vi "本地数字信号仿真 - 副本.vi"() -> ()   [LabVIEW 2012]
uses:
  <vilib>/ptbypt/Frequency Domain.llb/Real FFT PtByPt.vi
  <vilib>/ptbypt/NI_PtbyPt.lvlib
  <vilib>/Analysis/NI_AALBase.lvlib
panel:
  out "Last Element Inserted 3.78MHz":dbl caption="最后插入的元素" format="%0.2f"
  out "Last Element Removed 3.78MHz":dbl caption="最后删除的元素" format="%0.2f"
  out "Last Element Inserted":dbl caption="最后插入的元素" format="%0.2f"
  out "Last Element Removed":dbl caption="最后删除的元素" format="%0.2f"
  out "Elements in Queue":i32(slide) caption="队列中的元素" scale=0.0..60000000.0 scale format="%0.0f"
  out "Waveform Chart":cluster{"Last Element Inserted":dbl, dbl}(graph) caption="波形图表"
  out "Elements in Queue 2":i32(slide) caption="队列中的元素" scale=0.0..60000000.0 scale format="%0.0f"
  out "Waveform Chart 2":cluster{"Last Element Inserted":dbl, dbl}(graph) caption="波形图表"
  in  "Queue Size":i32=60000000 caption="队列大小"
  in  "停止":bool
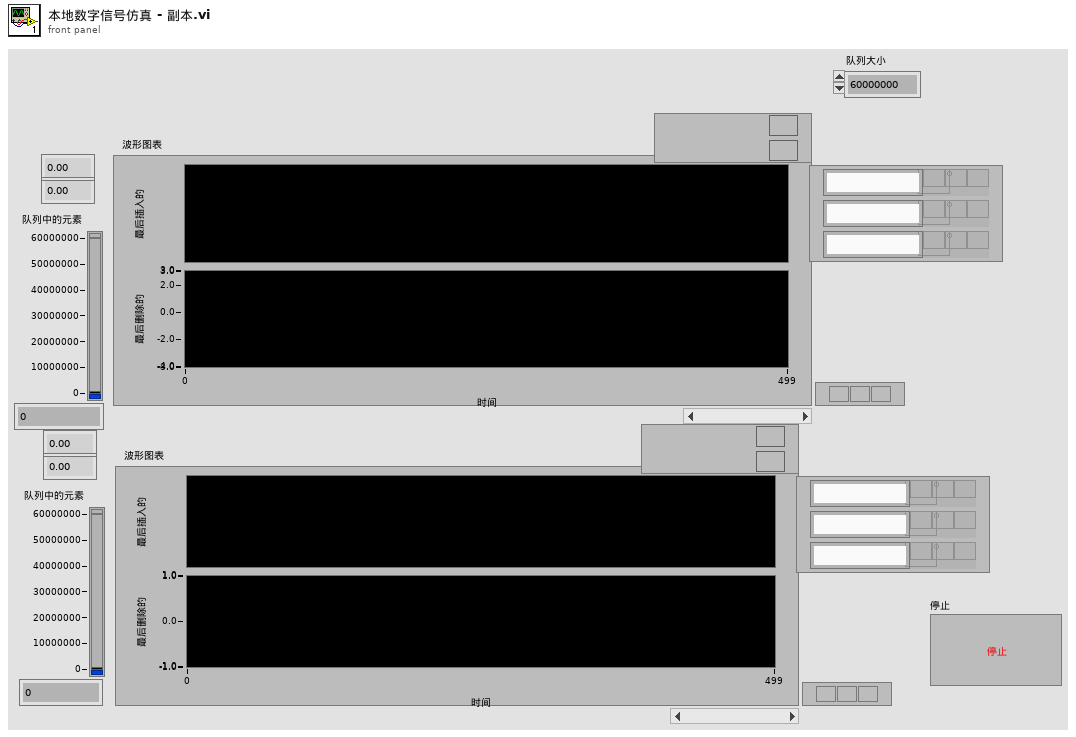
[diagram p1: front panel]
types:
  T1 = cluster{"Last Element Inserted":dbl, "Last Element Removed":dbl}
  T2 = cluster{"Last Element Inserted 3.78MHz":dbl, "Last Element Removed 3.78MHz":dbl}
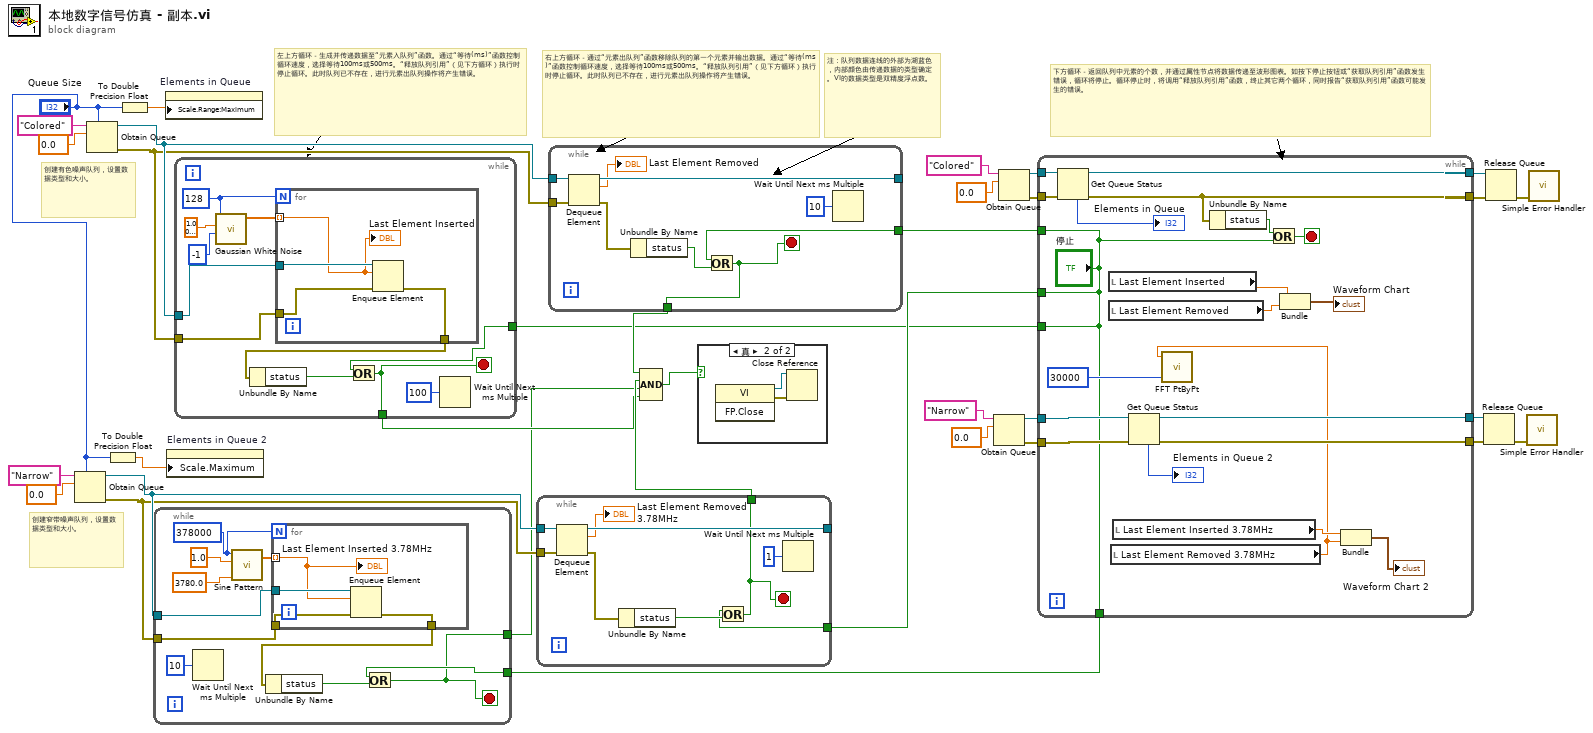
[diagram p0: block diagram]
diagram:
  # "创建窄带噪声队列，设置数据类型和大小。"
  # "右上方循环－通过“元素出队列”函数移除队列的第一个元素并输出数据。通过“等待(ms)”函数控制循环速度，选择等待100ms或500ms。“释放队列引用”（见下方循环）执行时停止循环。此时队列已不存在，进行元素出队列操作将产生错误。"
  # "注：队列数据连线的外部为湖蓝色，内部颜色由传递数据的类型确定。VI的数据类型是双精度浮点数。"
  # "下方循环－返回队列中元素的个数，并通过属性节点将数据传递至波形图表。如按下停止按钮或“获取队列引用”函数发生错误，循环将停止。循环停止时，将调用“释放队列引用”函数，终止其它两个循环，同时报告“获取队列引用”函数可能发生的错误。"
  # "左上方循环－生成并传递数据至“元素入队列”函数。通过“等待(ms)”函数控制循环速度，选择等待100ms或500ms。“释放队列引用”（见下方循环）执行时停止循环。此时队列已不存在，进行元素出队列操作将产生错误。"
  # "创建有色噪声队列，设置数据类型和大小。"
  n1 = Obtain Queue(max queue size (-1, unlimited)="Queue Size", name (unnamed)="Narrow", element data type=0.0) -> (queue out=w22:refnum<queue>, error out=w21:errorcluster)  [unwired: 2 in, 1 out]
  n2 = Obtain Queue(max queue size (-1, unlimited)="Queue Size", name (unnamed)="Colored", element data type=0.0) -> (queue out=w26:refnum<queue>, error out=w25:errorcluster)  [unwired: 2 in, 1 out]
  n3 = To Double Precision Float(number="Queue Size") -> (double precision float=w20:dbl)
  n4 = To Double Precision Float(number="Queue Size") -> (double precision float=w34:dbl)
  n5 = property on="Elements in Queue" class="Slide (严格)"("Scale.Range:Maximum"=w34) -> ()  [unwired: 2 in, 2 out]
  n6 = property on="Elements in Queue 2" class="Slide (严格)"("Scale.Maximum"=w20) -> ()  [unwired: 2 in, 2 out]
  n7 = Obtain Queue(name (unnamed)="Narrow", element data type=0.0) -> (queue out=w13:refnum<queue>, error out=w12:errorcluster)  [unwired: 3 in, 1 out]
  n8 = Obtain Queue(name (unnamed)="Colored", element data type=0.0) -> (queue out=w28:refnum<queue>, error out=w27:errorcluster)  [unwired: 3 in, 1 out]
  n9 = while {
    tunnel: w28 -> [w54]
    tunnel: [w47] -> w31
    tunnel: w27 -> [w50]
    tunnel: [w48] -> w30
    tunnel: w13 -> [w41]
    tunnel: w12 -> [w40]
    tunnel: [w39] -> w11
    tunnel: [w38] -> w10
    tunnel: ["停止"] -> w6
    tunnel: ["停止"] -> w5
    tunnel: ["停止"] -> w4
    tunnel: ["停止"] -> w3
    stop <- w52 stop-if-true
    n10 = Get Queue Status(queue=w54, error in (no error)=w50) -> (queue out=w48:refnum<queue>, error out=w47:errorcluster, # elements in queue=→"Elements in Queue":i32)  [unwired: 6 out]
    n11 = local read "Last Element Inserted"() -> (w49:dbl)
    n12 = local read "Last Element Removed"() -> (w45:dbl)
    n13 = local read "Last Element Removed 3.78MHz"() -> (w36:dbl)
    n14 = local read "Last Element Inserted 3.78MHz"() -> (w43:dbl)
    n15 = Get Queue Status(queue=w41, error in (no error)=w40) -> (queue out=w39:refnum<queue>, error out=w38:errorcluster, # elements in queue=→"Elements in Queue 2":i32)  [unwired: 6 out]
    n16 = call-poly <vilib>:"FFT PtByPt.vi"("sample length"=30000, "x"=w36) -> ()  [unwired: 2 in, 2 out]
    n17 = Unbundle By Name(w47) -> ("status"=w51:bool)
    n18 = Or(x=w51, y="停止") -> (x .or. y?=w52:bool)
    n19 = Bundle("Last Element Inserted"=w49, "Last Element Removed"=w45) -> (→"Waveform Chart":T1)  [unwired: 1 out]
    n20 = Bundle("Last Element Inserted 3.78MHz"=w43, "Last Element Removed 3.78MHz"=w36) -> (→"Waveform Chart 2":T2)  [unwired: 1 out]
  }
  n21 = while {
    tunnel: w22 -> [w65]
    tunnel: w21 -> [w64]
    tunnel: w3 -> [w56]
    tunnel: [w55] -> w1
    stop <- w55 stop-if-true
    w59 = 378000 ("samples")
    n22 = Wait Until Next ms Multiple(millisecond multiple=u32 10 ("milliseconds to wait")) -> ()  [unwired: 1 out]
    n23 = call <vilib>:"Sine Pattern.vi"("cycles"=3780.0, "amplitude"=1.0, "samples"=w59) -> ("Sinusoidal Pattern"=w60:dbl[])  [unwired: 1 in, 1 out]
    n24 = for {
      N: w59 -> [_]
      tunnel: w65 -> [w69]
      tunnel: w64 -> [w68]
      tunnel: [w67] -> w57
      tunnel: w60 -> [w66] mode=indexing
      n25 = Enqueue Element(queue=w69, element=w66, error in (no error)=w68) -> (error out=w67:errorcluster)  [unwired: 3 out]
      "Last Element Inserted 3.78MHz" <- w66
    }
    n26 = Unbundle By Name(w57) -> ("status"=w58:bool)
    n27 = Or(x=w56, y=w58) -> (x .or. y?=w55:bool)
  }
  n28 = while {
    tunnel: w26 -> [w77]
    tunnel: w25 -> [w76]
    tunnel: w4 -> [w71]
    tunnel: [w70] -> w2
    stop <- w70 stop-if-true
    w78 = 128 ("samples")
    n29 = call <vilib>:"Gaussian White Noise.vi"("seed"=-1, "standard deviation"=1.0000000000000002, "samples"=w78) -> ("Gaussian noise pattern"=w75:dbl[])  [unwired: 7 in, 1 out]
    n30 = for {
      N: w78 -> [_]
      tunnel: [w84] -> w72
      tunnel: w77 -> [w83]
      tunnel: w76 -> [w82]
      tunnel: w75 -> [w81] mode=indexing
      n31 = Enqueue Element(queue=w83, element=w81, error in (no error)=w82) -> (error out=w84:errorcluster)  [unwired: 3 out]
      "Last Element Inserted" <- w81
    }
    n32 = Unbundle By Name(w72) -> ("status"=w73:bool)
    n33 = Or(x=w71, y=w73) -> (x .or. y?=w70:bool)
    n34 = Wait Until Next ms Multiple(millisecond multiple=u32 100 ("milliseconds to wait")) -> ()  [unwired: 1 out]
  }
  n35 = while {
    tunnel: w22 -> [w93]
    tunnel: [w92] -> _
    tunnel: w21 -> [w91]
    tunnel: [w86] -> w7
    tunnel: w5 -> [w85]
    stop <- w86 stop-if-true
    n36 = Dequeue Element(queue=w93, error in (no error)=w91) -> (queue out=w92:refnum<queue>, element=→"Last Element Removed 3.78MHz":dbl, error out=w88:errorcluster)  [unwired: 2 out]
    n37 = Unbundle By Name(w88) -> ("status"=w87:bool)
    n38 = Or(x=w85, y=w87) -> (x .or. y?=w86:bool)
    n39 = Wait Until Next ms Multiple(millisecond multiple=u32 1 ("milliseconds to wait")) -> ()  [unwired: 1 out]
  }
  n40 = while {
    tunnel: w26 -> [w102]
    tunnel: [w101] -> _
    tunnel: w25 -> [w100]
    tunnel: [w95] -> w9
    tunnel: w6 -> [w94]
    stop <- w95 stop-if-true
    n41 = Dequeue Element(queue=w102, error in (no error)=w100) -> (queue out=w101:refnum<queue>, element=→"Last Element Removed":dbl, error out=w97:errorcluster)  [unwired: 2 out]
    n42 = Unbundle By Name(w97) -> ("status"=w96:bool)
    n43 = Or(x=w94, y=w96) -> (x .or. y?=w95:bool)
    n44 = Wait Until Next ms Multiple(millisecond multiple=u32 10 ("milliseconds to wait")) -> ()  [unwired: 1 out]
  }
  n45 = Compound Arithmetic op=AND(w9, w7, w1, w2) -> (w8:bool)
  n46 = case shown="真" w8 {
    frame False {
    }
    frame True {
      n47 = invoke class="VI" method="FP.Close"() -> (reference out=w103:refnum<vi>, error out=w104:errorcluster)  [unwired: 3 in, 1 out]
      n48 = Close Reference(reference=w103, error in (no error)=w104) -> ()  [unwired: 1 out]
    }
  }
  n49 = Release Queue(queue=w11, error in (no error)=w10) -> (error out=w14:errorcluster)  [unwired: 3 out]
  n50 = Release Queue(queue=w30, error in (no error)=w31) -> (error out=w18:errorcluster)  [unwired: 3 out]
  n51 = call <vilib>:"Simple Error Handler.vi"("error in (no error)"=w14) -> ()  [unwired: 1 in, 8 out]
  n52 = call <vilib>:"Simple Error Handler.vi"("error in (no error)"=w18) -> ()  [unwired: 1 in, 8 out]
